vi "TA_Plot_3DSurface_1.vi"() -> ()   [LabVIEW 2025]
uses:
  <vilib>/Math Plots/3D Math Plots/3D Surface/3D Surface XCtrl/3D Surface.xctl
  TA_DATA.ctl
  <vilib>/Math Plots/3D Math Plots/3D Surface/3D Surface Datatype/Public/Plot Helper (Vector).vi
  <vilib>/Math Plots/3D Math Plots/3D Surface/3D Surface Datatype/3D Surface Datatype.lvclass
panel:
  out "TA Data":T1
  out "TA 3D Surface":refnum<class "3D Plot Datatype.lvclass">[](xcontrol)
  in  "File Path":path=path "\\\\Mac\\Home/Desktop/fs-TA/Data/demo_fsta.dat"
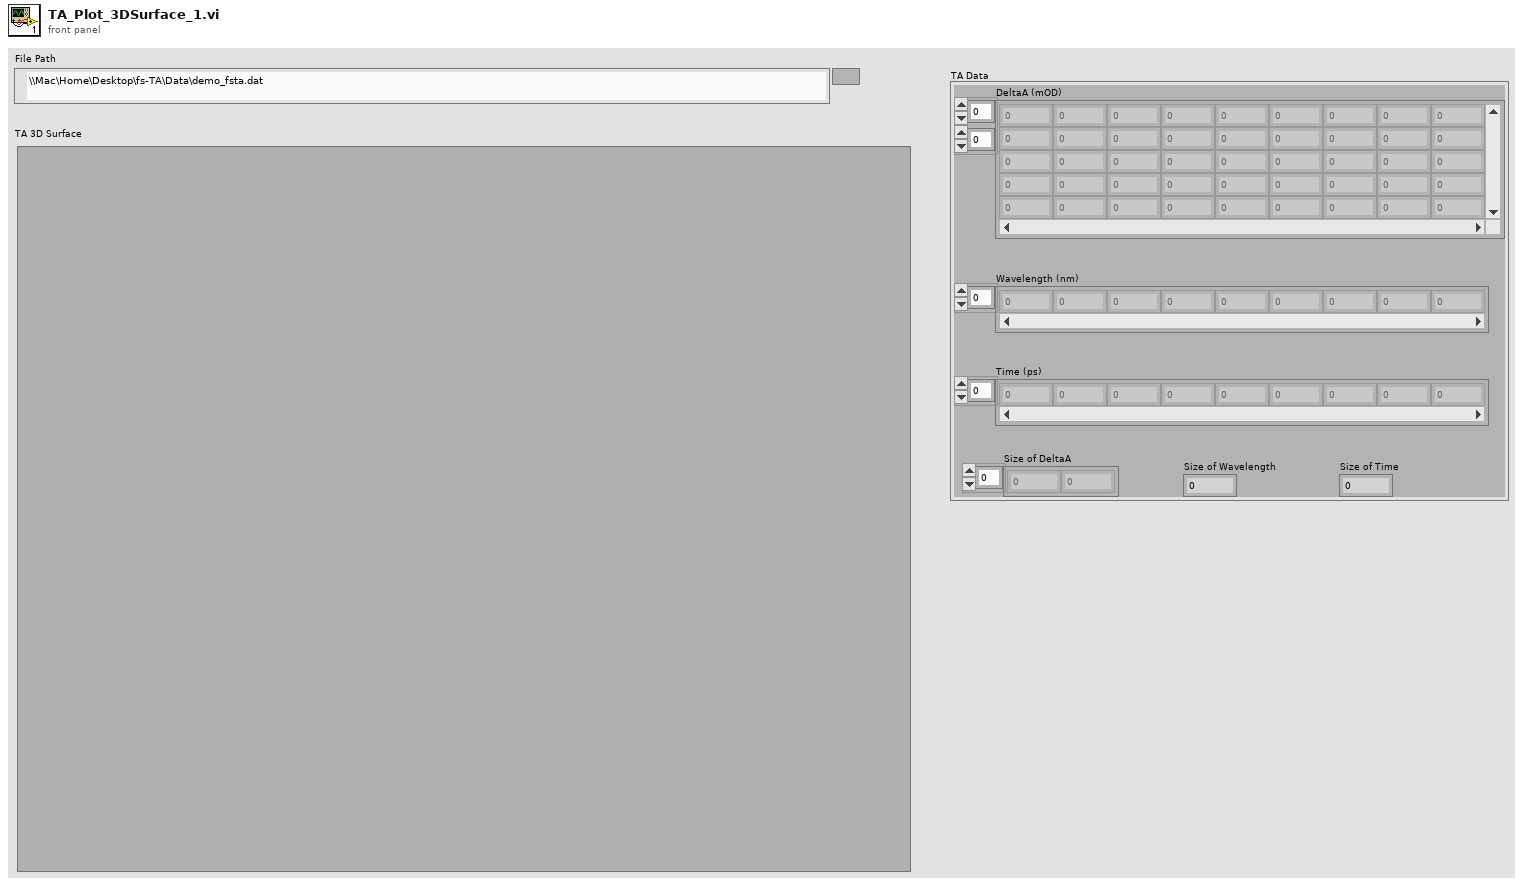
[diagram p1: front panel]
types:
  T1 = typedef "TA_DATA.ctl" = cluster{"DeltaA (mOD)":dbl[][], "Wavelength (nm)":dbl[], "Time (ps)":dbl[], "Size of DeltaA":i32[], "Size of Wavelength":i32, "Size of Time":i32}
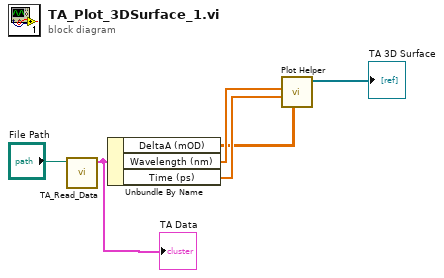
[diagram p0: block diagram]
diagram:
  n1 = call "TA_Read_Data.vi"("File Path"="File Path") -> ("TA Data"=w1:T1)  [unwired: 10 in]
  "TA Data" <- w1
  n2 = Unbundle By Name(w1) -> ("DeltaA (mOD)"=w2:dbl[][], "Wavelength (nm)"=w4:dbl[], "Time (ps)"=w3:dbl[])
  n3 = call-poly <vilib>:"Plot Helper.vi"("z matrix"=w2, "y vector"=w3, "x vector"=w4) -> ("3D Plot lvclass Array out"=→"TA 3D Surface":refnum<class "3D Plot Datatype.lvclass">[])  [unwired: 3 in, 5 out]
